vi "Compare Calls.vi"(8 "error in (no error)":errorcluster, 9 "VI Call 2":refnum<class "VI Call.lvclass">, 10 "VI Call 1":refnum<class "VI Call.lvclass">, 11 "Identical Inputs Comparator In":refnum<class "Identical Inputs Comparator.lvclass">) -> (0 "error out":errorcluster, 1 "Description":string, 2 "Equal?":bool)   [LabVIEW 2020, in "Identical Inputs Comparator.lvclass"]
uses:
  Identical Inputs Comparator.lvclass
  Core/VI Call/VI Call.lvclass
  Describe Comparison.vi
  <vilib>/AdvancedString/1D String Array to Delimited String.vi
  Core/Comparator/Describe Variant.vi
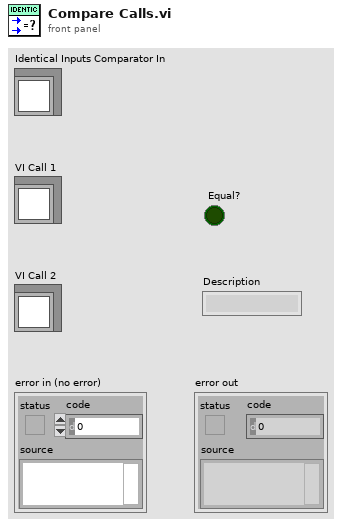
[diagram p1: front panel]
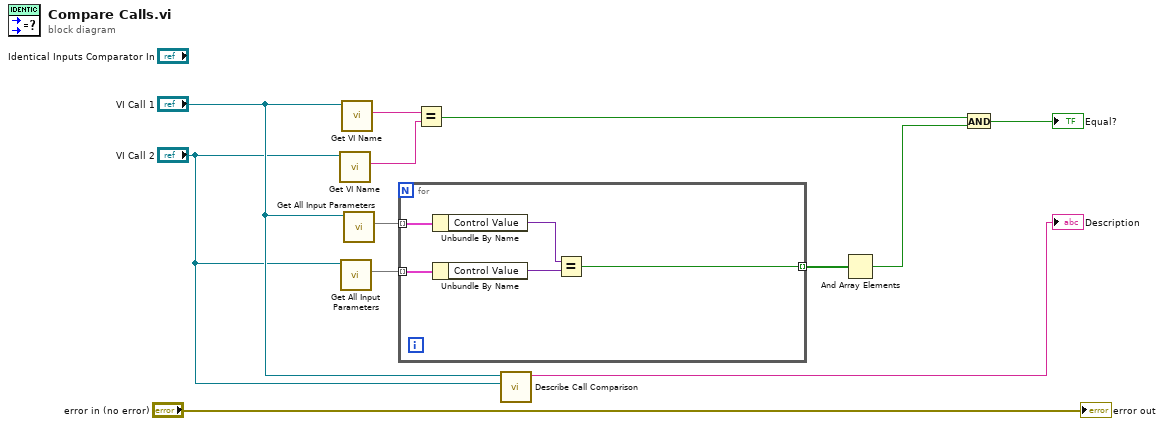
[diagram p0: block diagram]
diagram:
  n1 = call-dynamic "Get VI Name.vi"("VI Call In"="VI Call 2") -> ("VI Name"=w11:string)  [unwired: 9 in, 1 out]
  n2 = call-dynamic "Get All Input Parameters.vi"("VI Call in"="VI Call 2") -> ("Input Parameters"=w8:map{string, variant})  [unwired: 9 in, 1 out]
  n3 = call-dynamic "Get VI Name.vi"("VI Call In"="VI Call 1") -> ("VI Name"=w12:string)  [unwired: 9 in, 1 out]
  n4 = call-dynamic "Get All Input Parameters.vi"("VI Call in"="VI Call 1") -> ("Input Parameters"=w9:map{string, variant})  [unwired: 9 in, 1 out]
  n5 = for {
    tunnel: w9 -> [w17] mode=indexing
    tunnel: w8 -> [w16] mode=indexing
    tunnel: [w13] -> w7 mode=indexing
    n6 = Unbundle By Name(w17) -> ("Control Value"=w15:variant)
    n7 = Unbundle By Name(w16) -> ("Control Value"=w14:variant)
    n8 = Equal?(x=w15, y=w14) -> (x = y?=w13:bool)
  }
  n9 = Equal?(x=w12, y=w11) -> (x = y?=w5:bool)
  n10 = call "Describe Call Comparison.vi"("VI Call 2"="VI Call 2", "VI Call in"="VI Call 1") -> ("delimited string"=→"Description":string)  [unwired: 9 in]
  n11 = And Array Elements(Boolean array=w7) -> (logical AND=w6:bool)
  n12 = And(x=w5, y=w6) -> (x .and. y?=→"Equal?":bool)
  "error out" <- "error in (no error)"
